vi "Data Queue VI Tree.vi"   [LabVIEW 2016]
uses:
  Global Var.vi
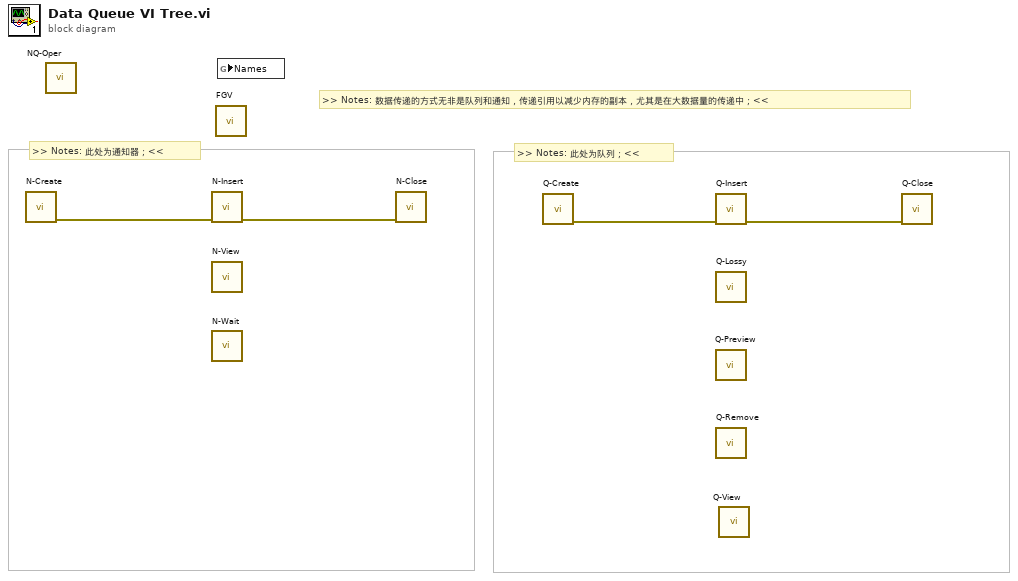
[diagram p0: block diagram]
diagram:
  # ">> Notes: 数据传递的方式无非是队列和通知，传递引用以减少内存的副本，尤其是在大数据量的传递中；<<"
  # ">> Notes: 此处为队列；<<"
  # ">> Notes: 此处为通知器；<<"
  n1 = call "N-Create.vi"() -> ("error out"=w4:errorcluster)  [unwired: 11 in]
  n2 = call-poly "NQ-Oper.vi"() -> ()  [unwired: 11 in, 1 out]
  n3 = call "N-Insert.vi"("error in"=w4) -> ("error out"=w3:errorcluster)  [unwired: 10 in]
  n4 = call "N-View.vi"() -> ()  [unwired: 10 in, 2 out]
  n5 = call "N-Wait.vi"() -> ()  [unwired: 9 in, 3 out]
  n6 = call "FGV.vi"() -> ()  [unwired: 7 in, 5 out]
  n7 = global read "Global Var.vi" "Names"() -> ()  [unwired: 1 in]
  n8 = call "N-Close.vi"("error in"=w3) -> ()  [unwired: 10 in, 1 out]
  n9 = call "Q-Create.vi"() -> ("error out"=w2:errorcluster)  [unwired: 11 in]
  n10 = call "Q-Insert.vi"("error in"=w2) -> ("error out"=w1:errorcluster)  [unwired: 10 in]
  n11 = call "Q-Lossy.vi"() -> ()  [unwired: 11 in, 1 out]
  n12 = call "Q-Preview.vi"() -> ()  [unwired: 6 in, 6 out]
  n13 = call "Q-Remove.vi"() -> ()  [unwired: 6 in, 6 out]
  n14 = call "Q-View.vi"() -> ()  [unwired: 7 in, 5 out]
  n15 = call "Q-Close.vi"("error in"=w1) -> ()  [unwired: 10 in, 1 out]
